vi "图形与图片.vi"() -> ()   [LabVIEW 2012]
uses:
  <vilib>/measure/mamon.llb/Waveform Peak Detection for 1 Chan.vi
  <vilib>/Waveform/WDTOps.llb/WDT Get XY Value DBL.vi
  PictureBox/Picture Box Tools.lvlib
  <vilib>/measure/NI_MAPro.lvlib
  <vilib>/measure/NI_MABase.lvlib
panel:
  out "波形图":waveform(dbl)(graph)
  in  "stop":bool
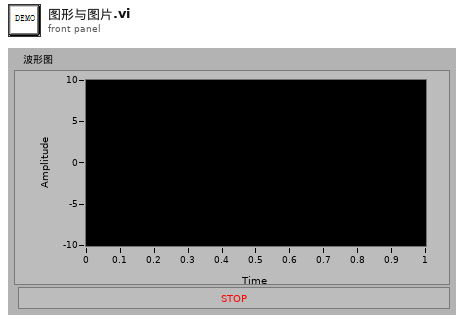
[diagram p1: front panel]
types:
  T1 = cluster{"绘图区域:大小:高度":u32, "绘图区域:大小:高度":u32, "Width":u32, "Height":u32}
  T2 = typedef "LVRectTypeDef.ctl" = cluster{"Left":i16, "Top":i16, "Right":i16, "Bottom":i16}
  T3 = typedef "LVPoint32TypeDef.ctl" = cluster{"Horizontal":i32, "Vertical":i32}
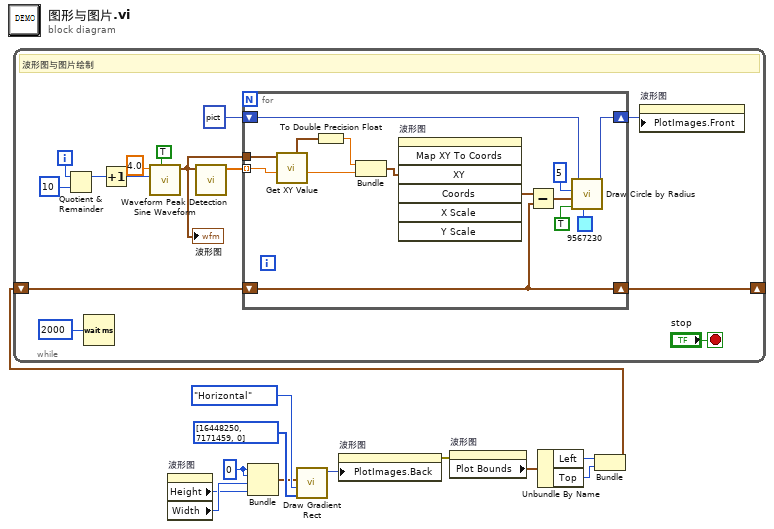
[diagram p0: block diagram]
diagram:
  w9 = u32 0 ("绘图区域:大小:高度")
  n1 = property on="波形图" class="WFGraph (严格)"() -> ("Height"=w7:u32, "Width"=w8:u32)  [unwired: 2 in, 2 out]
  n2 = Bundle("绘图区域:大小:高度"=w9, "绘图区域:大小:高度"=w9, "Width"=w8, "Height"=w7) -> (w6:T1)  [unwired: 1 in]
  n3 = call "Draw Gradient Rect.vi"("Color Segement"=u32[] [16448250, 7171459, 0], "Mode"=enum16{"Horizontal", "Vertical"}."Horizontal", "rect"=w6) -> ("picture out"=w10:picture)  [unwired: 8 in]
  n4 = property on="波形图" class="WFGraph (严格)"("PlotImages.Back"=w10) -> (error out=w1:errorcluster)  [unwired: 2 in, 1 out]
  n5 = property on="波形图" class="WFGraph (严格)"(error in=w1) -> ("Plot Bounds"=w3:T2)  [unwired: 1 in, 2 out]
  n6 = Unbundle By Name(w3) -> ("Left"=w5:i16, "Top"=w4:i16)
  n7 = Bundle("Left"=w5, "Top"=w4) -> (w2:cluster{"Left":i16, "Top":i16})  [unwired: 1 in]
  n8 = while "While循环" {
    shift-right: [w14] -> _
    shift-left: w2 -> [w15]
    i -> [w18]
    stop <- "stop" stop-if-true
    # "波形图与图片绘制"
    n9 = Quotient & Remainder(x=w18, y=10) -> (x-y*floor(x/y)=w17:i32)  [unwired: 1 out]
    n10 = Wait (ms)(milliseconds to wait=u32 2000 ("等待时间（毫秒）")) -> ()  [unwired: 1 out]
    n11 = Increment(x=w17) -> (x+1=w16:i32)
    n12 = call <vilib>:"Sine Waveform.vi"("reset signal"=TRUE, "amplitude"=w16, "frequency"=4.0) -> ("signal out"=w22:waveform(dbl))  [unwired: 7 in, 1 out]
    "波形图" <- w22
    n13 = call-poly <vilib>:"Waveform Peak Detection.vi"("Signal In"=w22) -> ("Locations"=w23:dbl[])  [unwired: 6 in, 4 out]
    n14 = for {
      tunnel: w23 -> [w40] mode=indexing
      tunnel: w22 -> [w39]
      shift-right: [w31] -> w13
      shift-left: picture data[5B] ("曲线图像:中间") -> [w34]
      shift-right: [w27] -> w14
      shift-left: w15 -> [w27]
      n15 = call-poly <vilib>:"Get XY Value.vi"("Y position"=w40, "waveform in"=w39) -> ("Y value"=w36:dbl, "X value"=w38:timestamp)  [unwired: 5 in, 3 out]
      n16 = To Double Precision Float(number=w38) -> (double precision float=w37:dbl)
      n17 = Bundle(w37, "Y value"=w36) -> (w35:cluster{dbl, "Y value":dbl})  [unwired: 1 in]
      n18 = invoke on="波形图" class="WFGraph (严格)" method="Map XY To Coords"("XY"=w35) -> ("Coords"=w30:T3)  [unwired: 6 in, 6 out]
      n19 = Subtract(x=w30, y=w27) -> (x-y=w29:T3)
      n20 = call <vilib>:"Draw Circle by Radius.vi"("color(black)"=u32 9567230, "fill?(F)"=TRUE, "pixel center"=w29, "radius"=i16 5, "picture"=w34) -> ("new picture"=w31:picture)  [unwired: 6 in]
    }
    n21 = property on="波形图" class="WFGraph (严格)"("PlotImages.Front"=w13) -> ()  [unwired: 2 in, 2 out]
  }
